vi "Pipe Var Intf - Test.vi"() -> ()   [LabVIEW 2020, in "GOLPI library.lvlib"]
uses:
  GOLPI library.lvlib
  Public/GOLPI reference Type Def.ctl
  LV Process source distribution/Pipe Handle.ctl
  LV Process source distribution/LV Process library.lvlib
panel:
  in  "N":i32
  in  "M":i32
  in  "btn gen rand":bool
  out "time [s]":dbl format="%#_3p"
  out "write cycle":i32
  in  "write count":i32
  in  "btn cmd":bool
  in  "command":string
  in  "variable name":string
  in  "data":dbl[][](array[numeric])
  in  "btn write":bool
  in  "btn exit":bool
  out "GOLPI ref. out":T1={"pipe handle"={"lv_proc.dll file path"=path "", "process instance handle"=[], "debug mode"=FALSE, "debug data"=[]}, "fast read timeout [ms]"=500, "fast read settle time [ms]"=10, "fast read to multiple [ms]"=1, "max elements per input line"=100, "slow read timeout [ms]"=500, "stdin double format specifier"="", "max elements per stdout output column"=100, "console mode bitstream"=FALSE, "bitstream first read timeout [ms]"=1000, "bitstream read timeout [ms]"=50, "struct transfer possible"=FALSE, "matlab mode"=FALSE, "var pipe write timeout [ms]"=5000, "variable pipe mode"=FALSE, "variable pipe buffer size [Bytes]"=10000000, "variable pipe block size [Bytes]"=1000000} {"variable pipe block size [Bytes]" format="%.0p"; "variable pipe buffer size [Bytes]" format="%.0p"}
  in  "btn stop":bool
  in  "btn start":bool
  in  "working dir (user home)":path=path "F:/GOLPI/develop/golpi_pipes"
  in  "octave binary file or dir (autofind)":path=path "C:/Octave/Octave-4.2.2/bin/octave-cli.exe"
  out "error out":errorcluster
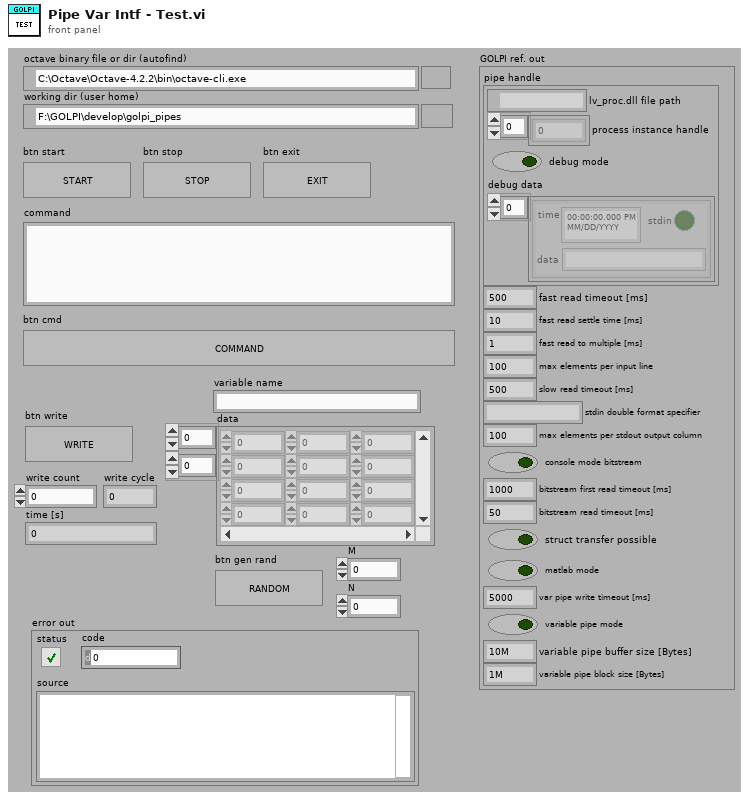
[diagram p1: front panel]
types:
  T1 = typedef "GOLPI library.lvlib/GOLPI reference Type Def.ctl" = cluster{"pipe handle":T2, "fast read timeout [ms]":u32, "fast read settle time [ms]":u32, "fast read to multiple [ms]":u32, "max elements per input line":u32, "slow read timeout [ms]":u32, "stdin double format specifier":string, "max elements per stdout output column":u32, "console mode bitstream":bool, "bitstream first read timeout [ms]":u32, "bitstream read timeout [ms]":u32, "struct transfer possible":bool, "matlab mode":bool, "var pipe write timeout [ms]":u32, "variable pipe mode":bool, "variable pipe buffer size [Bytes]":u32, "variable pipe block size [Bytes]":u32}
  T2 = typedef "LV Process library.lvlib/Pipe Handle.ctl" = cluster{"lv_proc.dll file path":path, "process instance handle":u32[], "debug mode":bool, "debug data":cluster{"time":timestamp, "stdin":bool, "data":string}[]}
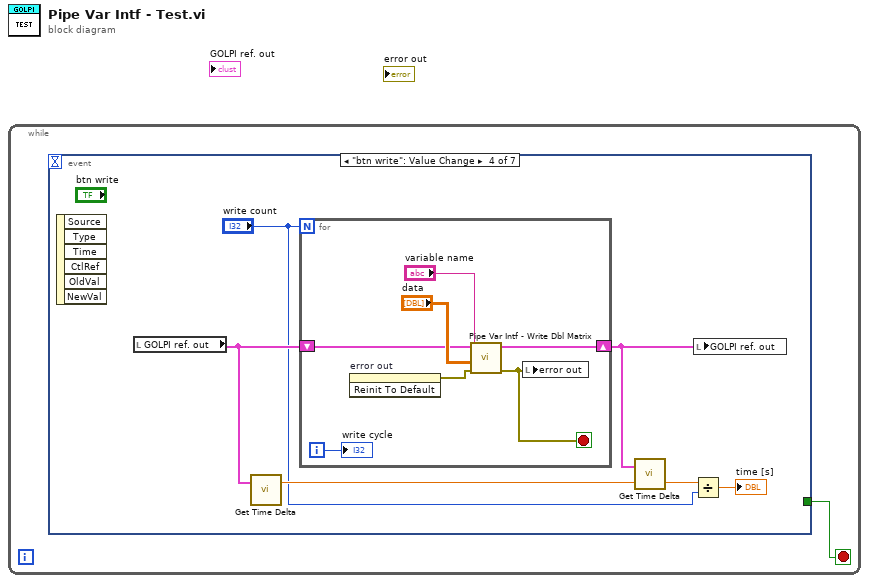
[diagram p0: block diagram]
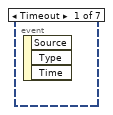
[diagram p2: hidden frame]
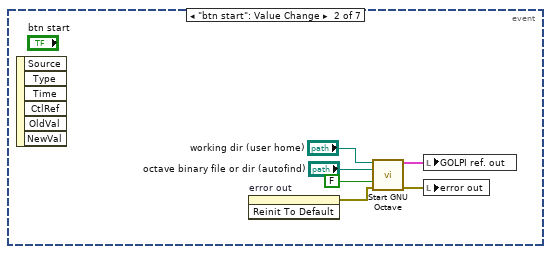
[diagram p3: hidden frame]
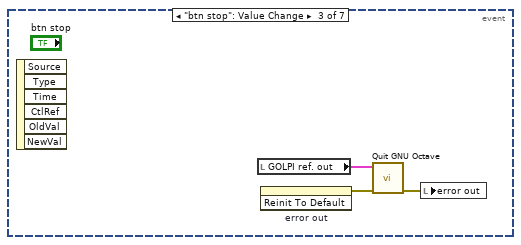
[diagram p4: hidden frame]
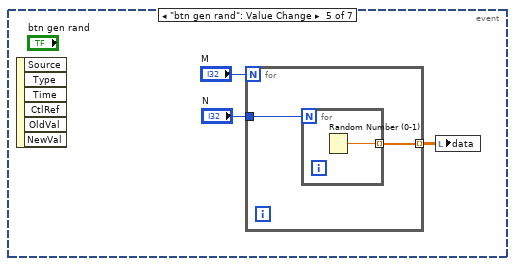
[diagram p5: hidden frame]
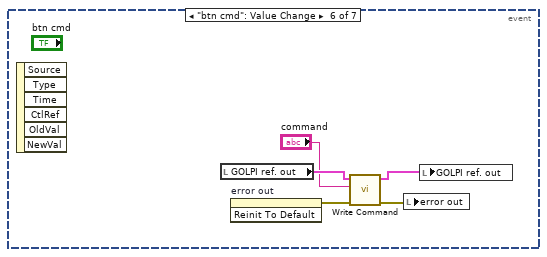
[diagram p6: hidden frame]
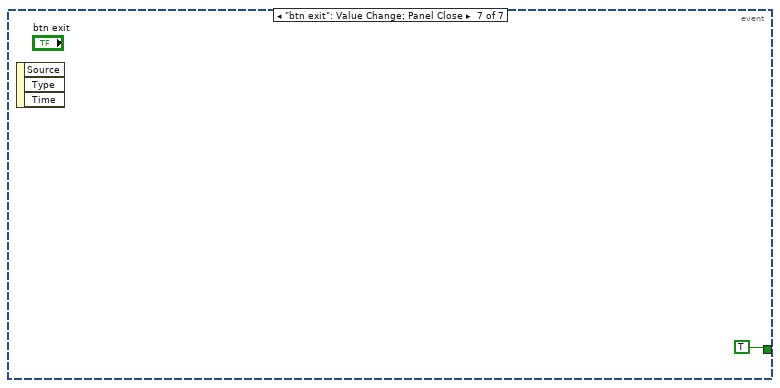
[diagram p7: hidden frame]
diagram:
  n1 = while {
    stop <- w1 stop-if-true
    n2 = event shown="[3] \"btn write\": Value Change" {
      selector: _ -> [_ _ _ _ _ _ _]
      dyn-events: _ -> [_ _ _ _ _ _ _]
      timeout: _ -> [_ _ _ _ _ _ _]
      tunnel: [_ _ _ _ _ _ TRUE] -> w1
      event Timeout {
        n3 = event-data() -> ()  [unwired: 1 in, 3 out]
      }
      event "btn start": Value Change {
        n4 = event-data() -> ()  [unwired: 1 in, 6 out]
        n5 = invoke on="error out" class="Clust (strict)" method="Reinit To Default"() -> (error out=w4:errorcluster)  [unwired: 3 in, 2 out]
        n6 = call "Start GNU Octave.vi"("working dir (user home)"="working dir (user home)", "octave binary file or dir (autofind)"="octave binary file or dir (autofind)", "hide debug console (T)"=FALSE, "error in"=w4) -> ("GOLPI ref. out"=w2:T1, "error out"=w3:errorcluster)  [unwired: 8 in, 2 out]
        n7 = local write "GOLPI ref. out"(w2) -> ()
        n8 = local write "error out"(w3) -> ()
      }
      event "btn stop": Value Change {
        n9 = event-data() -> ()  [unwired: 1 in, 6 out]
        n10 = local read "GOLPI ref. out"() -> (w10:T1)
        n11 = invoke on="error out" class="Clust (strict)" method="Reinit To Default"() -> (error out=w9:errorcluster)  [unwired: 3 in, 2 out]
        n12 = call "Quit GNU Octave.vi"("error in"=w9, "GOLPI ref. in"=w10) -> ("error out"=w8:errorcluster)  [unwired: 8 in, 1 out]
        n13 = local write "error out"(w8) -> ()
      }
      event "btn write": Value Change {
        n14 = event-data() -> ()  [unwired: 1 in, 6 out]
        n15 = local read "GOLPI ref. out"() -> (w16:T1)
        n16 = call "Get Time Delta.vi"("anything in (for synchronization)"=w16) -> ("time now"=w14:dbl)  [unwired: 1 in, 1 out]
        n17 = for {
          N: "write count" -> [_]
          shift-right: [w18] -> w15
          shift-left: w16 -> [w20]
          i -> [w19]
          stop <- w17 stop-if-true
          n18 = invoke on="error out" class="Clust (strict)" method="Reinit To Default"() -> (error out=w23:errorcluster)  [unwired: 3 in, 2 out]
          n19 = call "Pipe Var Intf - Write Dbl Matrix.vi"("error in (no error)"=w23, "data"="data", "variable name"="variable name", "GOLPI ref. in"=w20) -> ("error out"=w17:errorcluster, "GOLPI ref. out"=w18:T1)  [unwired: 6 in]
          n20 = local write "error out"(w17) -> ()
          "write cycle" <- w19
        }
        n21 = call "Get Time Delta.vi"("reference time (0)"=w14, "anything in (for synchronization)"=w15) -> ("time delta [s]"=w13:dbl)  [unwired: 1 out]
        n22 = Divide(x=w13, y="write count") -> (x/y=→"time [s]":dbl)
        n23 = local write "GOLPI ref. out"(w15) -> ()
      }
      event "btn gen rand": Value Change {
        n24 = event-data() -> ()  [unwired: 1 in, 6 out]
        n25 = for {
          N: "M" -> [_]
          tunnel: [w28] -> w26 mode=indexing
          tunnel: "N" -> [w27]
          n26 = for {
            N: w27 -> [_]
            tunnel: [w29] -> w28 mode=indexing
            n27 = Random Number (0-1)() -> (number: 0 to 1=w29:dbl)
          }
        }
        n28 = local write "data"(w26) -> ()
      }
      event "btn cmd": Value Change {
        n29 = event-data() -> ()  [unwired: 1 in, 6 out]
        n30 = local read "GOLPI ref. out"() -> (w32:T1)
        n31 = invoke on="error out" class="Clust (strict)" method="Reinit To Default"() -> (error out=w34:errorcluster)  [unwired: 3 in, 2 out]
        n32 = call "Write Command.vi"("error in"=w34, "command"="command", "GOLPI ref. in"=w32) -> ("error out"=w33:errorcluster, "GOLPI ref. out"=w31:T1)  [unwired: 7 in]
        n33 = local write "error out"(w33) -> ()
        n34 = local write "GOLPI ref. out"(w31) -> ()
      }
      event "btn exit": Value Change; Panel Close {
        n35 = event-data() -> ()  [unwired: 1 in, 3 out]
      }
    }
  }
